vi "LVJSON Merge.vi"(7 "Behavior (Add or Modify)":T1, 8 "error in (no error)":errorcluster, 10 "Element to Merge":T2, 11 "Root Element in":T2) -> (0 "error out":errorcluster, 2 "Exists?":bool, 3 "Root Element out":T2)   [LabVIEW 2019, in "labview_json.lvlib"]
uses:
  labview_json.lvlib
  Element.ctl
  Element Type.ctl
  Element Set Behavior.ctl
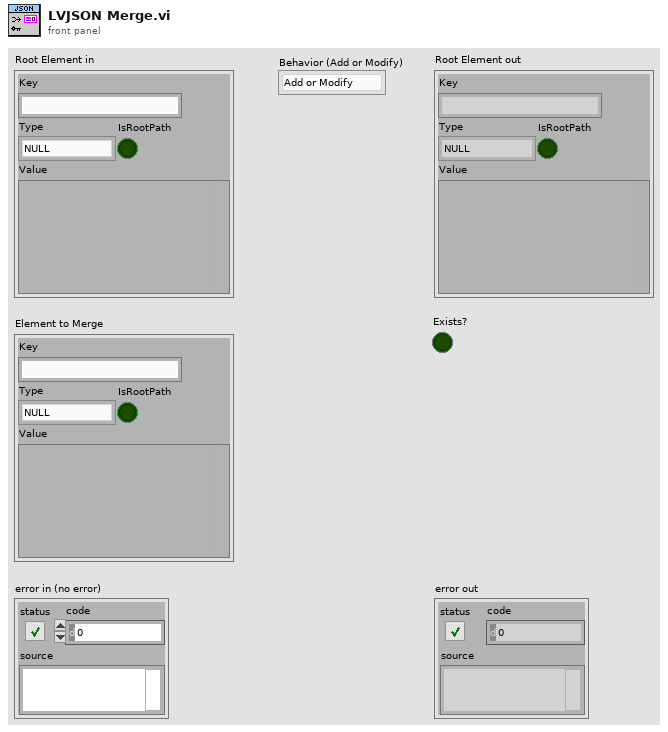
[diagram p1: front panel]
types:
  T1 = typedef "labview_json.lvlib/Element Set Behavior.ctl" = enum8{"Add or Modify", "Modify Only", "Replace"}
  T2 = typedef "labview_json.lvlib/Element.ctl" = cluster{"Key":string, "Type":T3, "Value":variant, "IsRootPath":bool}
  T3 = typedef "labview_json.lvlib/Element Type.ctl" = enum8{"NULL", "OBJECT", "ARRAY", "BOOL", "INT", "UINT", "FLOAT", "STRING"}
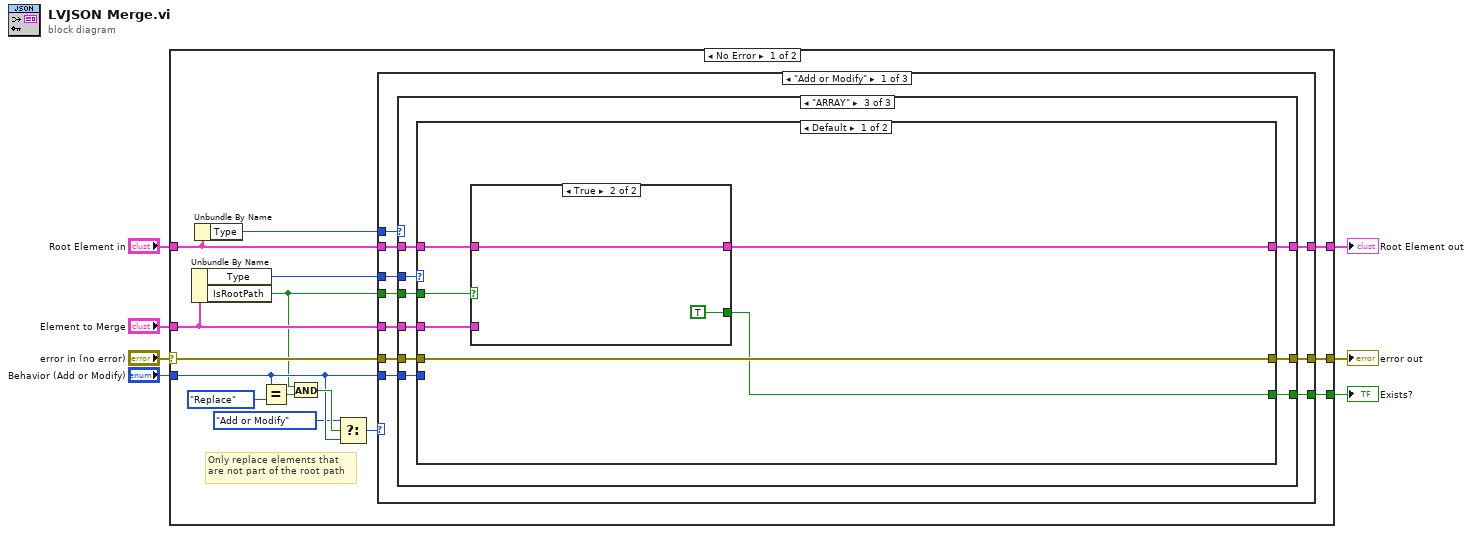
[diagram p0: block diagram]
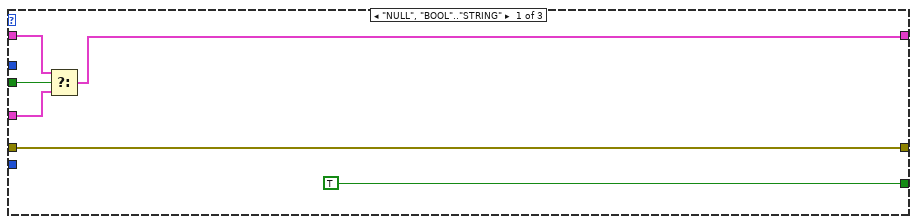
[diagram p2: hidden frame]
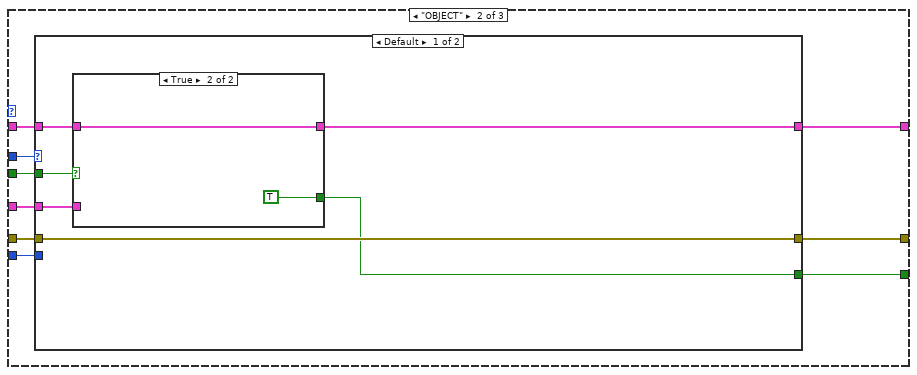
[diagram p3: hidden frame]
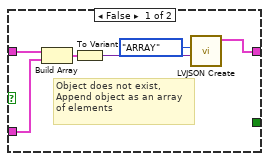
[diagram p4: hidden frame]
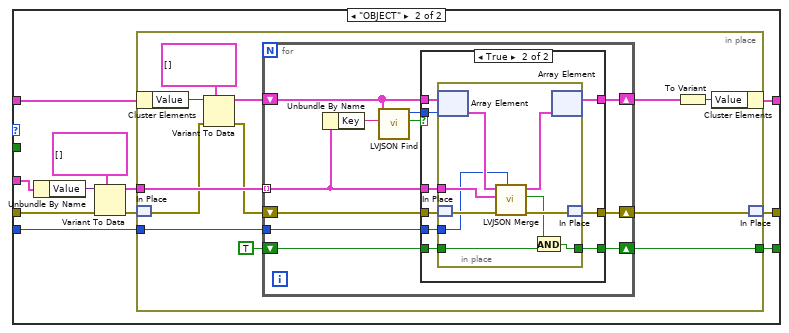
[diagram p5: hidden frame]
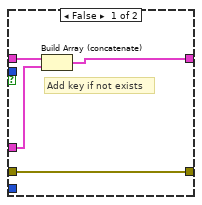
[diagram p6: hidden frame]
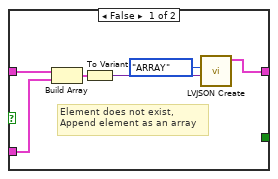
[diagram p7: hidden frame]
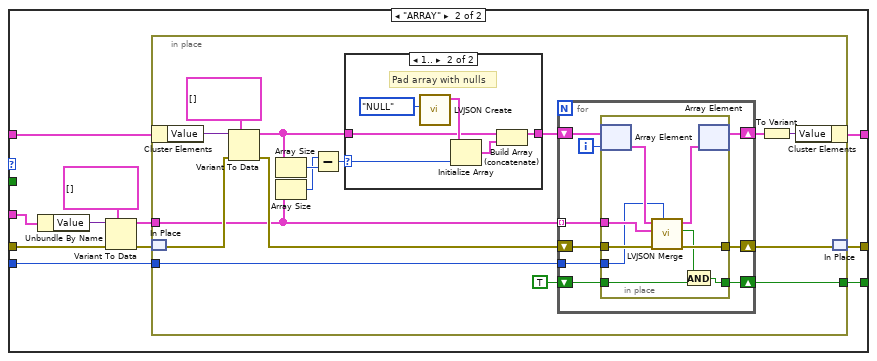
[diagram p8: hidden frame]
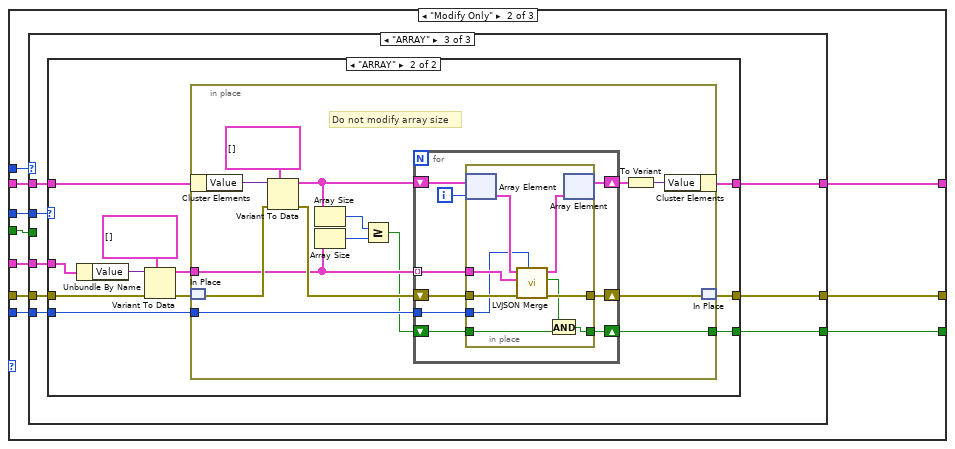
[diagram p10: hidden frame]
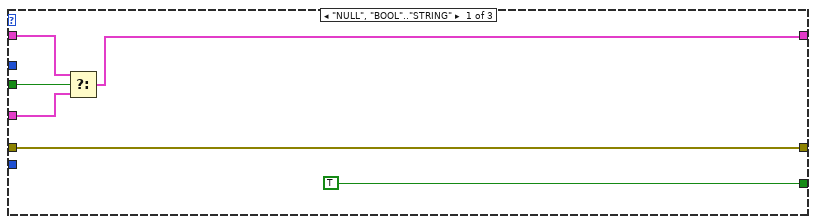
[diagram p11: hidden frame]
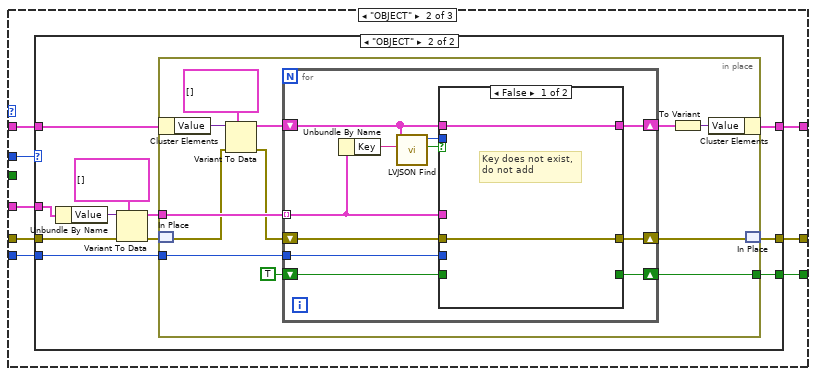
[diagram p12: hidden frame]
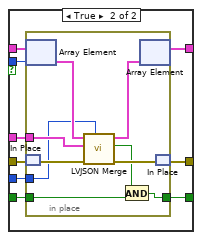
[diagram p14: hidden frame]
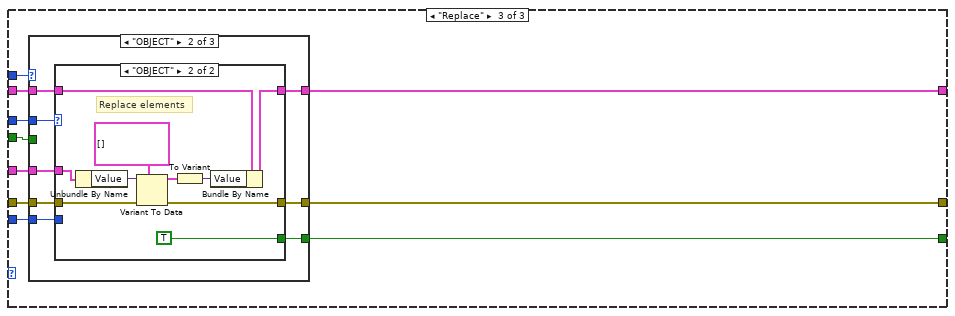
[diagram p16: hidden frame]
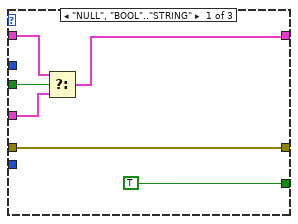
[diagram p17: hidden frame]
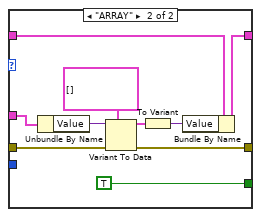
[diagram p20: hidden frame]
diagram:
  n1 = case shown="No Error" "error in (no error)" {
    selector: "error in (no error)" -> [w20 w383]
    tunnel: [w19 w383] -> w7
    tunnel: "Root Element in" -> [w22 w382]
    tunnel: "Element to Merge" -> [w9 _]
    tunnel: [w21 w382] -> w3
    tunnel: [w18 _] -> w2
    tunnel: "Behavior (Add or Modify)" -> [w13 _]
    frame No Error {
      # "Only replace elements that\nare not part of the root path"
      n2 = Unbundle By Name(w9) -> ("Type"=w10:T3, "IsRootPath"=w8:bool)
      n3 = Unbundle By Name(w22) -> ("Type"=w17:T3)
      n4 = Equal?(x=w13, y=Element_Set_Behavior."Replace") -> (x = y?=w15:bool)
      n5 = And(x=w8, y=w15) -> (x .and. y?=w14:bool)
      n6 = Select(t=Element_Set_Behavior."Add or Modify", s=w14, f=w13) -> (s? t:f=w11:T1)
      n7 = case shown="\"Add or Modify\"" w11 {
        tunnel: w22 -> [w32 w202 w335]
        tunnel: [w31 w201 w334] -> w21
        tunnel: w20 -> [w30 w200 w333]
        tunnel: [w29 w199 w332] -> w19
        tunnel: [w28 w198 w331] -> w18
        tunnel: w17 -> [w27 w197 w330]
        tunnel: w10 -> [w26 w196 w329]
        tunnel: w9 -> [w25 w195 w328]
        tunnel: w13 -> [w24 w194 w327]
        tunnel: w8 -> [w23 w193 w326]
        frame "Add or Modify" {
          n8 = case shown="\"ARRAY\"" w27 {
            tunnel: w32 -> [w35 w46 w126]
            tunnel: [w34 w44 w123] -> w31
            tunnel: w25 -> [w33 w42 w121]
            tunnel: w30 -> [w38 w47 w125]
            tunnel: [w38 w45 w124] -> w29
            tunnel: [TRUE ("Exists?") w43 w122] -> w28
            tunnel: w24 -> [_ w40 w120]
            tunnel: w26 -> [_ w41 w119]
            tunnel: w23 -> [w36 w39 w118]
            frame "NULL", "BOOL".."STRING" {
              n9 = Select(t=w35, s=w36, f=w33) -> (s? t:f=w34:T2)
            }
            frame "OBJECT" {
              n10 = case shown="Default" w41 {
                tunnel: w47 -> [w50 w66]
                tunnel: w46 -> [w53 w72]
                tunnel: [w50 w71] -> w45
                tunnel: [w51 w70] -> w44
                tunnel: [w48 w69] -> w43
                tunnel: w42 -> [w52 w65]
                tunnel: w40 -> [_ w62]
                tunnel: w39 -> [w49 _]
                frame Default {
                  n11 = case shown="True" w49 {
                    tunnel: w53 -> [w59 w61]
                    tunnel: w52 -> [w58 _]
                    tunnel: [w57 w61] -> w51
                    tunnel: [_ TRUE] -> w48
                    frame False {
                      # "Object does not exist,\nAppend object as an array\nof elements"
                      n12 = Build Array(w59, w58) -> (w55:T2[])
                      n13 = To Variant(anything=w55) -> (Variant=w54:variant)
                      n14 = call "LVJSON Create.vi"("Variant (Void=Default Type)"=w54, "Type"=Element_Type."ARRAY") -> ("Element out"=w57:T2)  [unwired: 9 in]
                    }
                    frame True {
                    }
                  }
                }
                frame "OBJECT" {
                  n15 = Unbundle By Name(w65) -> ("Value"=w64:variant)
                  n16 = Variant To Data(error in=w66, type=T2[] [], Variant=w64) -> (data=w63:T2[], error out=w67:errorcluster)
                  n17 = in-place {
                    in-place-border: w63 -> [w82]
                    in-place-border: [w76] -> w69
                    in-place-border: w62 -> [w74]
                    n18 = in-place-cluster #1(w72) -> ("Value"=w81:variant)
                    n19 = in-place-match #2(w67) -> (w79:errorcluster)
                    n20 = Variant To Data(error in=w79, type=T2[] [], Variant=w81) -> (data=w83:T2[], error out=w78:errorcluster)
                    n21 = for {
                      tunnel: w82 -> [w92] mode=indexing
                      shift-right: [w89] -> w77
                      shift-left: w78 -> [w90]
                      shift-right: [w93] -> w75
                      shift-left: w83 -> [w94]
                      shift-right: [w91] -> w76
                      shift-left: TRUE ("Exists?") -> [w87]
                      tunnel: w74 -> [w86]
                      n22 = Unbundle By Name(w92) -> ("Key"=w85:string)
                      n23 = call "LVJSON Find.vi"("Key"=w85, "Elements in"=w94) -> ("Found?"=w95:bool, "Index"=w88:i32)  [unwired: 8 in]
                      n24 = case shown="True" w95 {
                        tunnel: w94 -> [w99 w108]
                        tunnel: w88 -> [_ w107]
                        tunnel: w92 -> [w97 w103]
                        tunnel: [w98 w106] -> w93
                        tunnel: [_ w102] -> w91
                        tunnel: w90 -> [w96 w105]
                        tunnel: [w96 w104] -> w89
                        tunnel: w87 -> [_ w101]
                        tunnel: w86 -> [_ w100]
                        frame False {
                          # "Add key if not exists"
                          n25 = Build Array (concatenate)(w99, w97) -> (w98:T2[])
                        }
                        frame True {
                          n26 = in-place {
                            in-place-border: w103 -> [w116]
                            in-place-border: [w110] -> w102
                            in-place-border: w101 -> [w112]
                            in-place-border: w100 -> [w109]
                            n27 = in-place-array #3(w108, w107) -> (w115:T2)
                            n28 = in-place-match #4(w105) -> (w117:errorcluster)
                            n29 = call "LVJSON Merge.vi"("Behavior (Add or Modify)"=w109, "error in (no error)"=w117, "Element to Merge"=w116, "Root Element in"=w115) -> ("error out"=w113:errorcluster, "Exists?"=w111:bool, "Root Element out"=w114:T2)  [unwired: 5 in]
                            n30 = And(x=w111, y=w112) -> (x .and. y?=w110:bool)
                            n31 = in-place-array #3(w114) -> (w106:T2[])  [unwired: 1 out]
                            n32 = in-place-match #4(w113) -> (w104:errorcluster)
                          }
                        }
                      }
                    }
                    n33 = To Variant(anything=w75) -> (Variant=w80:variant)
                    n34 = in-place-cluster #1("Value"=w80) -> (w70:T2)
                    n35 = in-place-match #2(w77) -> (w71:errorcluster)
                  }
                }
              }
            }
            frame "ARRAY" {
              n36 = case shown="Default" w119 {
                tunnel: w126 -> [w132 w151]
                tunnel: w125 -> [w130 w150]
                tunnel: [w130 w149] -> w124
                tunnel: [w129 w148] -> w123
                tunnel: [w127 w147] -> w122
                tunnel: w121 -> [w131 w142]
                tunnel: w120 -> [_ w141]
                tunnel: w118 -> [w128 _]
                frame Default {
                  n37 = case shown="True" w128 {
                    tunnel: w132 -> [w138 w140]
                    tunnel: w131 -> [w137 _]
                    tunnel: [w136 w140] -> w129
                    tunnel: [_ TRUE] -> w127
                    frame False {
                      # "Element does not exist,\nAppend element as an array"
                      n38 = Build Array(w138, w137) -> (w134:T2[])
                      n39 = To Variant(anything=w134) -> (Variant=w133:variant)
                      n40 = call "LVJSON Create.vi"("Variant (Void=Default Type)"=w133, "Type"=Element_Type."ARRAY") -> ("Element out"=w136:T2)  [unwired: 9 in]
                    }
                    frame True {
                    }
                  }
                }
                frame "ARRAY" {
                  n41 = Unbundle By Name(w142) -> ("Value"=w145:variant)
                  n42 = Variant To Data(error in=w150, type=T2[] [], Variant=w145) -> (data=w143:T2[], error out=w146:errorcluster)
                  n43 = in-place {
                    in-place-border: w143 -> [w159]
                    in-place-border: [w163] -> w147
                    in-place-border: w141 -> [w157]
                    n44 = in-place-cluster #5(w151) -> ("Value"=w165:variant)
                    n45 = in-place-match #6(w146) -> (w164:errorcluster)
                    n46 = Variant To Data(error in=w164, type=T2[] [], Variant=w165) -> (data=w158:T2[], error out=w161:errorcluster)
                    n47 = Array Size(array=w158) -> (size(s)=w156:i32)
                    n48 = Array Size(array=w159) -> (size(s)=w155:i32)
                    n49 = Subtract(x=w155, y=w156) -> (x-y=w153:i32)
                    n50 = case shown="1.." w153 {
                      selector: w153 -> [_ w169]
                      tunnel: w158 -> [w168 w171]
                      tunnel: [w168 w170] -> w154
                      frame ..0 {
                      }
                      frame 1.. {
                        # "Pad array with nulls"
                        n51 = call "LVJSON Create.vi"("Type"=Element_Type."NULL") -> ("Element out"=w173:T2)  [unwired: 10 in]
                        n52 = Initialize Array(w173, w169) -> (w172:T2[])
                        n53 = Build Array (concatenate)(w171, w172) -> (w170:T2[])
                      }
                    }
                    n54 = for {
                      tunnel: w159 -> [w177] mode=indexing
                      shift-right: [w180] -> w160
                      shift-left: w161 -> [w181]
                      shift-right: [w179] -> w162
                      shift-left: w154 -> [w183]
                      shift-right: [w182] -> w163
                      shift-left: TRUE ("Exists?") -> [w176]
                      tunnel: w157 -> [w175]
                      i -> [w178]
                      n55 = in-place {
                        in-place-border: w181 -> [w192]
                        in-place-border: [w191] -> w180
                        in-place-border: [w185] -> w182
                        in-place-border: w177 -> [w188]
                        in-place-border: w176 -> [w186]
                        in-place-border: w175 -> [w184]
                        n56 = in-place-array #7(w183, w178) -> (w189:T2)
                        n57 = call "LVJSON Merge.vi"("Behavior (Add or Modify)"=w184, "error in (no error)"=w192, "Element to Merge"=w188, "Root Element in"=w189) -> ("error out"=w191:errorcluster, "Exists?"=w187:bool, "Root Element out"=w190:T2)  [unwired: 5 in]
                        n58 = And(x=w187, y=w186) -> (x .and. y?=w185:bool)
                        n59 = in-place-array #7(w190) -> (w179:T2[])  [unwired: 1 out]
                      }
                    }
                    n60 = To Variant(anything=w162) -> (Variant=w166:variant)
                    n61 = in-place-cluster #5("Value"=w166) -> (w148:T2)
                    n62 = in-place-match #6(w160) -> (w149:errorcluster)
                  }
                }
              }
            }
          }
        }
        frame "Modify Only" {
          n63 = case shown="\"ARRAY\"" w197 {
            tunnel: w202 -> [w205 w215 w280]
            tunnel: [w203 w213 w277] -> w201
            tunnel: w195 -> [w204 w211 w275]
            tunnel: w200 -> [w208 w216 w279]
            tunnel: [w208 w214 w278] -> w199
            tunnel: [TRUE ("Exists?") w212 w276] -> w198
            tunnel: w194 -> [_ w209 w274]
            tunnel: w196 -> [_ w210 w273]
            tunnel: w193 -> [w206 _ _]
            frame "NULL", "BOOL".."STRING" {
              n64 = Select(t=w205, s=w206, f=w204) -> (s? t:f=w203:T2)
            }
            frame "OBJECT" {
              n65 = case shown="\"OBJECT\"" w210 {
                tunnel: w216 -> [w218 w223]
                tunnel: w215 -> [w217 w229]
                tunnel: [w218 w228] -> w214
                tunnel: [w217 w227] -> w213
                tunnel: [_ w226] -> w212
                tunnel: w211 -> [_ w222]
                tunnel: w209 -> [_ w219]
                frame Default {
                  # "Object does not exist,\nDo not append"
                }
                frame "OBJECT" {
                  n66 = Unbundle By Name(w222) -> ("Value"=w221:variant)
                  n67 = Variant To Data(error in=w223, type=T2[] [], Variant=w221) -> (data=w220:T2[], error out=w224:errorcluster)
                  n68 = in-place {
                    in-place-border: w220 -> [w239]
                    in-place-border: [w233] -> w226
                    in-place-border: w219 -> [w231]
                    n69 = in-place-cluster #8(w229) -> ("Value"=w238:variant)
                    n70 = in-place-match #9(w224) -> (w236:errorcluster)
                    n71 = Variant To Data(error in=w236, type=T2[] [], Variant=w238) -> (data=w240:T2[], error out=w235:errorcluster)
                    n72 = for {
                      tunnel: w239 -> [w249] mode=indexing
                      shift-right: [w246] -> w234
                      shift-left: w235 -> [w247]
                      shift-right: [w250] -> w232
                      shift-left: w240 -> [w251]
                      shift-right: [w248] -> w233
                      shift-left: TRUE ("Exists?") -> [w244]
                      tunnel: w231 -> [w243]
                      n73 = Unbundle By Name(w249) -> ("Key"=w242:string)
                      n74 = call "LVJSON Find.vi"("Key"=w242, "Elements in"=w251) -> ("Found?"=w252:bool, "Index"=w245:i32)  [unwired: 8 in]
                      n75 = case shown="False" w252 {
                        tunnel: w251 -> [w253 w263]
                        tunnel: w245 -> [_ w262]
                        tunnel: w249 -> [_ w258]
                        tunnel: [w253 w261] -> w250
                        tunnel: [_ w257] -> w248
                        tunnel: w247 -> [w254 w260]
                        tunnel: [w254 w259] -> w246
                        tunnel: w244 -> [_ w256]
                        tunnel: w243 -> [_ w255]
                        frame False {
                          # "Key does not exist,\ndo not add"
                        }
                        frame True {
                          n76 = in-place {
                            in-place-border: w258 -> [w271]
                            in-place-border: [w265] -> w257
                            in-place-border: w256 -> [w267]
                            in-place-border: w255 -> [w264]
                            n77 = in-place-array #10(w263, w262) -> (w270:T2)
                            n78 = in-place-match #11(w260) -> (w272:errorcluster)
                            n79 = call "LVJSON Merge.vi"("Behavior (Add or Modify)"=w264, "error in (no error)"=w272, "Element to Merge"=w271, "Root Element in"=w270) -> ("error out"=w268:errorcluster, "Exists?"=w266:bool, "Root Element out"=w269:T2)  [unwired: 5 in]
                            n80 = And(x=w266, y=w267) -> (x .and. y?=w265:bool)
                            n81 = in-place-array #10(w269) -> (w261:T2[])  [unwired: 1 out]
                            n82 = in-place-match #11(w268) -> (w259:errorcluster)
                          }
                        }
                      }
                    }
                    n83 = To Variant(anything=w232) -> (Variant=w237:variant)
                    n84 = in-place-cluster #8("Value"=w237) -> (w227:T2)
                    n85 = in-place-match #9(w234) -> (w228:errorcluster)
                  }
                }
              }
            }
            frame "ARRAY" {
              n86 = case shown="\"ARRAY\"" w273 {
                tunnel: w280 -> [w281 w293]
                tunnel: w279 -> [w282 w292]
                tunnel: [w282 w291] -> w278
                tunnel: [w281 w290] -> w277
                tunnel: [_ w289] -> w276
                tunnel: w275 -> [_ w284]
                tunnel: w274 -> [_ w283]
                frame Default {
                  # "Array does not exist,\nDo not append"
                }
                frame "ARRAY" {
                  n87 = Unbundle By Name(w284) -> ("Value"=w287:variant)
                  n88 = Variant To Data(error in=w292, type=T2[] [], Variant=w287) -> (data=w285:T2[], error out=w288:errorcluster)
                  n89 = in-place {
                    in-place-border: w285 -> [w299]
                    in-place-border: [w303] -> w289
                    in-place-border: w283 -> [w298]
                    # "Do not modify array size"
                    n90 = in-place-cluster #12(w293) -> ("Value"=w305:variant)
                    n91 = in-place-match #13(w288) -> (w304:errorcluster)
                    n92 = Variant To Data(error in=w304, type=T2[] [], Variant=w305) -> (data=w297:T2[], error out=w301:errorcluster)
                    n93 = Array Size(array=w297) -> (size(s)=w296:i32)
                    n94 = Array Size(array=w299) -> (size(s)=w295:i32)
                    n95 = Greater Or Equal?(x=w296, y=w295) -> (x >= y?=w294:bool)
                    n96 = for {
                      tunnel: w299 -> [w310] mode=indexing
                      shift-right: [w313] -> w300
                      shift-left: w301 -> [w314]
                      shift-right: [w312] -> w302
                      shift-left: w297 -> [w316]
                      shift-right: [w315] -> w303
                      shift-left: w294 -> [w309]
                      tunnel: w298 -> [w308]
                      i -> [w311]
                      n97 = in-place {
                        in-place-border: w314 -> [w325]
                        in-place-border: [w324] -> w313
                        in-place-border: [w318] -> w315
                        in-place-border: w310 -> [w321]
                        in-place-border: w309 -> [w319]
                        in-place-border: w308 -> [w317]
                        n98 = in-place-array #14(w316, w311) -> (w322:T2)
                        n99 = call "LVJSON Merge.vi"("Behavior (Add or Modify)"=w317, "error in (no error)"=w325, "Element to Merge"=w321, "Root Element in"=w322) -> ("error out"=w324:errorcluster, "Exists?"=w320:bool, "Root Element out"=w323:T2)  [unwired: 5 in]
                        n100 = And(x=w320, y=w319) -> (x .and. y?=w318:bool)
                        n101 = in-place-array #14(w323) -> (w312:T2[])  [unwired: 1 out]
                      }
                    }
                    n102 = To Variant(anything=w302) -> (Variant=w306:variant)
                    n103 = in-place-cluster #12("Value"=w306) -> (w290:T2)
                    n104 = in-place-match #13(w300) -> (w291:errorcluster)
                  }
                }
              }
            }
          }
        }
        frame "Replace" {
          n105 = case shown="\"OBJECT\"" w330 {
            tunnel: w335 -> [w338 w348 w369]
            tunnel: [w337 w346 w366] -> w334
            tunnel: w328 -> [w336 w344 w364]
            tunnel: w333 -> [w341 w349 w368]
            tunnel: [w341 w347 w367] -> w332
            tunnel: [TRUE ("Exists?") w345 w365] -> w331
            tunnel: w327 -> [_ w342 w363]
            tunnel: w329 -> [_ w343 w362]
            tunnel: w326 -> [w339 _ _]
            frame "NULL", "BOOL".."STRING" {
              n106 = Select(t=w338, s=w339, f=w336) -> (s? t:f=w337:T2)
            }
            frame "OBJECT" {
              n107 = case shown="\"OBJECT\"" w343 {
                tunnel: w349 -> [w351 w358]
                tunnel: w348 -> [_ w361]
                tunnel: [w351 w354] -> w347
                tunnel: [w350 w360] -> w346
                tunnel: [_ TRUE ("Exists?")] -> w345
                tunnel: w344 -> [w350 w357]
                tunnel: w342 -> [_ _]
                frame Default {
                  # "Object does not exist,\nReplace element"
                }
                frame "OBJECT" {
                  # "Replace elements"
                  n108 = Unbundle By Name(w357) -> ("Value"=w356:variant)
                  n109 = Variant To Data(error in=w358, type=T2[] [], Variant=w356) -> (data=w352:T2[], error out=w354:errorcluster)
                  n110 = To Variant(anything=w352) -> (Variant=w355:variant)
                  n111 = Bundle By Name(cluster=w361, "Value"=w355) -> (w360:T2)
                }
              }
            }
            frame "ARRAY" {
              n112 = case shown="Default" w362 {
                tunnel: w369 -> [_ w377]
                tunnel: w368 -> [w371 w381]
                tunnel: [w371 w372] -> w367
                tunnel: [w370 w375] -> w366
                tunnel: [_ TRUE] -> w365
                tunnel: w364 -> [w370 w378]
                tunnel: w363 -> [_ _]
                frame Default {
                  # "Array does not exist,\nReplace element"
                }
                frame "ARRAY" {
                  n113 = Unbundle By Name(w378) -> ("Value"=w380:variant)
                  n114 = Variant To Data(error in=w381, type=T2[] [], Variant=w380) -> (data=w374:T2[], error out=w372:errorcluster)
                  n115 = To Variant(anything=w374) -> (Variant=w373:variant)
                  n116 = Bundle By Name(cluster=w377, "Value"=w373) -> (w375:T2)
                }
              }
            }
          }
        }
      }
    }
    frame Error {
    }
  }
  "error out" <- w7
  "Exists?" <- w2
  "Root Element out" <- w3
